vi "FT10_FPGA_7854R Set Config.vi"(11 "7854 Config Enum":T1) -> (0 "Config string":string="LigaSure", 1 "Conn2/DIO_16_23 In":bool[](array[boolean]), 2 "Conn2/DIO_8_15 In":bool[](array[boolean]), 3 "Conn2/DIO_0_7 In":bool[](array[boolean]))   [LabVIEW 2024]
doc: "Sets the correct relays to be on for the specificied configuration."
uses:
  Controls/Control_PXI-7854R Set Config Enum.ctl
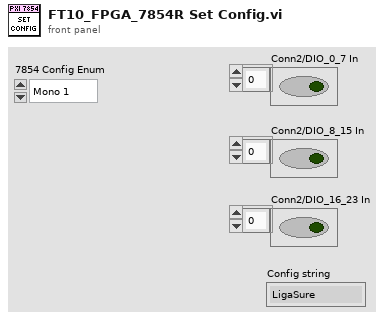
[diagram p1: front panel]
types:
  T1 = typedef "Control_PXI-7854R Set Config Enum.ctl" = enum16{"Mono 1", "Mono 2", "BiPolar", "LigaSure", "Off"}
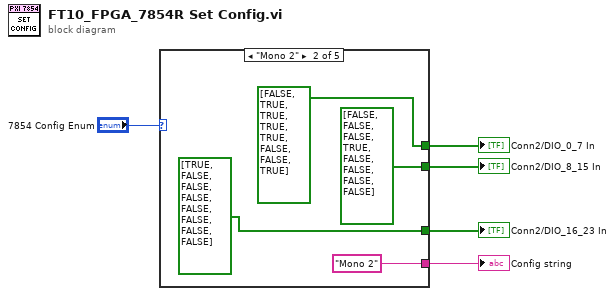
[diagram p0: block diagram]
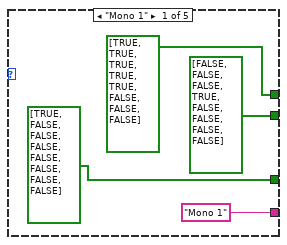
[diagram p2: hidden frame]
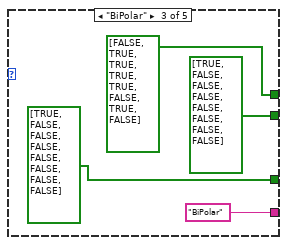
[diagram p3: hidden frame]
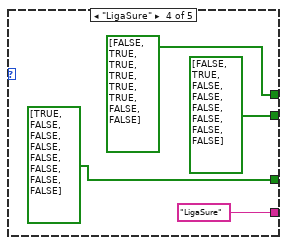
[diagram p4: hidden frame]
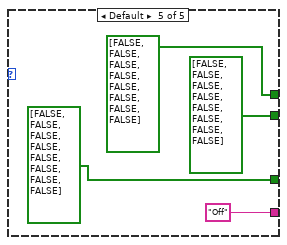
[diagram p5: hidden frame]
diagram:
  n1 = case shown="\"Mono 2\"" "7854 Config Enum" {
    tunnel: [bool[] [TRUE, TRUE, TRUE, TRUE, TRUE, FALSE, FALSE, FALSE] ("Conn2/DIO_0_7 In") bool[] [FALSE, TRUE, TRUE, TRUE, TRUE, FALSE, FALSE, TRUE] ("Conn2/DIO_0_7 In") bool[] [FALSE, TRUE, TRUE, TRUE, TRUE, FALSE, TRUE, FALSE] ("Conn2/DIO_0_7 In") bool[] [FALSE, TRUE, TRUE, TRUE, TRUE, TRUE, FALSE, FALSE] ("Conn2/DIO_0_7 In") bool[] [FALSE, FALSE, FALSE, FALSE, FALSE, FALSE, FALSE, FALSE] ("Conn2/DIO_0_7 In")] -> w4
    tunnel: [bool[] [FALSE, FALSE, FALSE, TRUE, FALSE, FALSE, FALSE, FALSE] ("Conn2/DIO_8_15 In") bool[] [FALSE, FALSE, FALSE, TRUE, FALSE, FALSE, FALSE, FALSE] ("Conn2/DIO_8_15 In") bool[] [TRUE, FALSE, FALSE, FALSE, FALSE, FALSE, FALSE, FALSE] ("Conn2/DIO_8_15 In") bool[] [FALSE, TRUE, FALSE, FALSE, FALSE, FALSE, FALSE, FALSE] ("Conn2/DIO_8_15 In") bool[] [FALSE, FALSE, FALSE, FALSE, FALSE, FALSE, FALSE, FALSE] ("Conn2/DIO_8_15 In")] -> w5
    tunnel: ["Mono 1" "Mono 2" "BiPolar" "LigaSure" "Off"] -> w3
    tunnel: [bool[] [TRUE, FALSE, FALSE, FALSE, FALSE, FALSE, FALSE, FALSE] ("Conn2/DIO_0_7 In") bool[] [TRUE, FALSE, FALSE, FALSE, FALSE, FALSE, FALSE, FALSE] ("Conn2/DIO_0_7 In") bool[] [TRUE, FALSE, FALSE, FALSE, FALSE, FALSE, FALSE, FALSE] ("Conn2/DIO_0_7 In") bool[] [TRUE, FALSE, FALSE, FALSE, FALSE, FALSE, FALSE, FALSE] ("Conn2/DIO_0_7 In") bool[] [FALSE, FALSE, FALSE, FALSE, FALSE, FALSE, FALSE, FALSE] ("Conn2/DIO_0_7 In")] -> w1
    frame "Mono 1" {
    }
    frame "Mono 2" {
    }
    frame "BiPolar" {
    }
    frame "LigaSure" {
    }
    frame Default {
    }
  }
  "Conn2/DIO_8_15 In" <- w5
  "Conn2/DIO_0_7 In" <- w4
  "Config string" <- w3
  "Conn2/DIO_16_23 In" <- w1
